vi "Day03-03.vi"() -> ()   [LabVIEW 2021]
panel:
  out "알람 경고 2":bool
  in  "알람 경고":bool
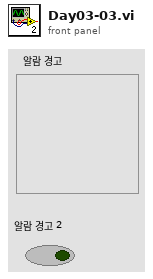
[diagram p1: front panel]
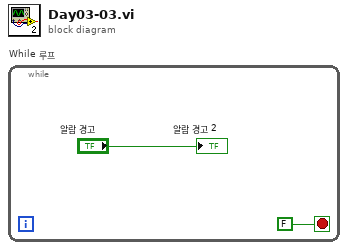
[diagram p0: block diagram]
diagram:
  n1 = while "While 루프" {
    stop <- FALSE stop-if-true
    "알람 경고 2" <- "알람 경고"
  }
